vi "字符串解包.vi"(11 "data out":string) -> (3 "数组":i32[][](array[numeric]))   [LabVIEW 2020]
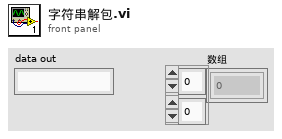
[diagram p1: front panel]
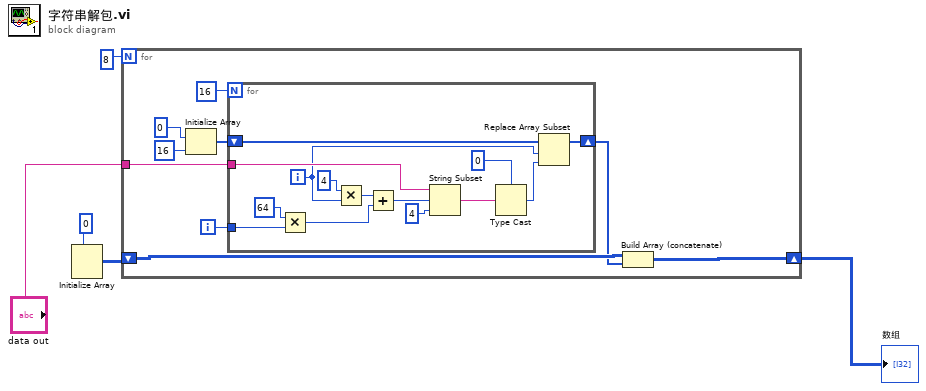
[diagram p0: block diagram]
diagram:
  n1 = Initialize Array(0) -> (w2:i32[][])  [unwired: 2 in]
  n2 = for {
    N: u16 8 -> [_]
    tunnel: "data out" -> [w14]
    shift-right: [w7] -> w5
    shift-left: w2 -> [w8]
    i -> [w9]
    n3 = Initialize Array(0, 16) -> (w10:i32[])
    n4 = for {
      N: i8 16 -> [_]
      tunnel: w14 -> [w26]
      tunnel: w9 -> [w22]
      shift-right: [w15] -> w6
      shift-left: w10 -> [w16]
      i -> [w17]
      n5 = Multiply(x=i8 64, y=w22) -> (x*y=w21:i32)
      n6 = Multiply(x=i8 4, y=w17) -> (x*y=w19:i32)
      n7 = Add(x=w19, y=w21) -> (x+y=w20:i32)
      n8 = String Subset(string=w26, offset (0)=w20, length (rest)=i8 4) -> (substring=w28:string)
      n9 = Type Cast(type=0, x=w28) -> (*(type *) &x=w18:i32)
      n10 = Replace Array Subset(array=w16, new element=w18, index=w17) -> (w15:i32[])
    }
    n11 = Build Array (concatenate)(w8, w6) -> (w7:i32[][])
  }
  "数组" <- w5
